vi "Check For Latched Booleans.vi"(8 "error in":errorcluster, 11 "path of type":path) -> (0 "error out":errorcluster, 3 "path of type out":path)   [LabVIEW 2020, in "MeasurementLink Measurement Server.lvlib"]
uses:
  MeasurementLink Measurement Server.lvlib
  Helpers/Error Strings Global Internal.vi
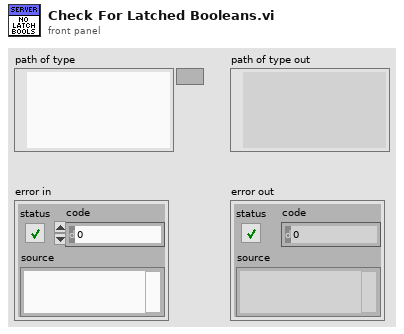
[diagram p1: front panel]
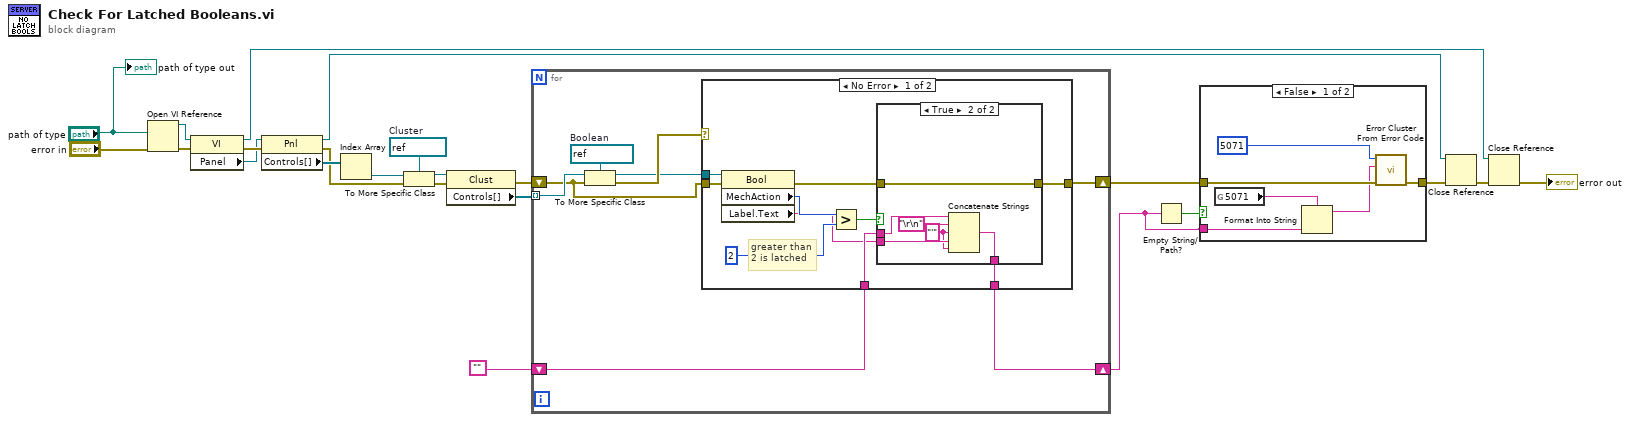
[diagram p0: block diagram]
diagram:
  w23 = refnum<vi> refnum  # Cluster
  n1 = Open VI Reference(vi path="path of type", error in (no error)="error in") -> (vi reference=w11:refnum<vi>, error out=w18:errorcluster)  [unwired: 4 in]
  n2 = property class="VI"(reference=w11, error in=w18) -> (reference out=w15:refnum<vi>, error out=w17:errorcluster, "Panel"=w12:refnum<vi>)
  n3 = property class="Pnl"(reference=w12, error in=w17) -> (reference out=w14:refnum<vi>, error out=w8:errorcluster, "Controls[]"=w13:refnum<vi>[])
  n4 = Index Array(array=w13) -> (element=w10:refnum<vi>)  [unwired: 1 in]
  n5 = To More Specific Class(target class=w23, reference=w10, error in=w8) -> (specific class reference=w22:refnum<vi>, error out=w20:errorcluster)
  n6 = property class="Clust"(reference=w22, error in=w20) -> (error out=w19:errorcluster, "Controls[]"=w21:refnum<vi>[])  [unwired: 1 out]
  n7 = for {
    tunnel: w21 -> [w31] mode=indexing
    shift-right: [w26] -> w5
    shift-left: w19 -> [w27]
    shift-right: [w24] -> w1
    shift-left: "" -> [w25]
    w30 = refnum<vi> refnum  # Boolean
    n8 = To More Specific Class(target class=w30, reference=w31, error in=w27) -> (specific class reference=w28:refnum<vi>, error out=w29:errorcluster)
    n9 = case shown="No Error" w29 {
      tunnel: w28 -> [w41 _]
      tunnel: w27 -> [w36 w51]
      tunnel: [w37 w51] -> w26
      tunnel: w25 -> [w34 w50]
      tunnel: [w32 w50] -> w24
      frame No Error {
        # "greater than\n2 is latched"
        n10 = property class="Bool"(reference=w41, error in=w36) -> (error out=w35:errorcluster, "MechAction"=w40:u32, "Label.Text"=w33:string)  [unwired: 1 out]
        n11 = Greater?(x=w40, y=u32 2) -> (0:w38:bool)
        n12 = case shown="True" w38 {
          tunnel: [w43 w49] -> w37
          tunnel: w35 -> [w43 w49]
          tunnel: w34 -> [w42 w47]
          tunnel: w33 -> [_ w45]
          tunnel: [w42 w48] -> w32
          frame False {
          }
          frame True {
            w44 = "'" ("string")
            n13 = Concatenate Strings(w47, "\r\n", w44, w45, w44) -> (w48:string)
          }
        }
      }
      frame Error {
      }
    }
  }
  n14 = Empty String/Path?(string/path=w1) -> (empty?=w2:bool)
  n15 = case shown="False" w2 {
    tunnel: w5 -> [w56 w58]
    tunnel: [w55 w58] -> w4
    tunnel: w1 -> [w53 _]
    frame False {
      n16 = global read "Error Strings Global Internal.vi" "5071"() -> (w54:string)
      n17 = Format Into String(format string=w54, w53) -> (resulting string=w52:string)  [unwired: 2 in, 1 out]
      n18 = call <vilib>:"Error Cluster From Error Code.vi"("error in (no error)"=w56, "error message (\"\")"=w52, "error code (0)"=5071) -> ("error out"=w55:errorcluster)  [unwired: 6 in]
    }
    frame True {
    }
  }
  n19 = Close Reference(reference=w14, error in (no error)=w4) -> (error out=w16:errorcluster)
  n20 = Close Reference(reference=w15, error in (no error)=w16) -> (error out=→"error out":errorcluster)
  "path of type out" <- "path of type"
